vi "activateBtnIHM.vi"(8 "error in (no error)":errorcluster, 10 "State":T1(ring), 11 "References":T2) -> (0 "error out":errorcluster)   [LabVIEW 2023]
uses:
  referencesBtns.ctl
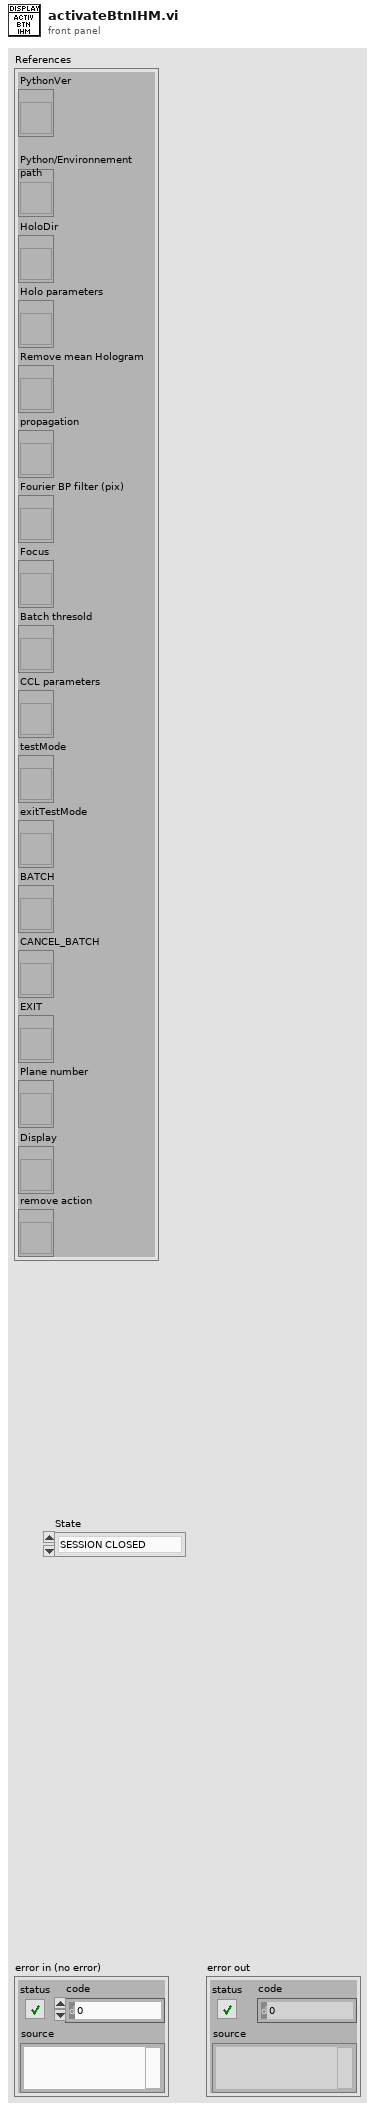
[diagram p1: front panel]
types:
  T1 = enum16{"SESSION CLOSED", "WAIT", "TEST WAIT", "TEST IN PROGESS", "BATCH IN PROGRESS"}
  T2 = typedef "referencesBtns.ctl" = cluster{"PythonVer":refnum<vi>, "Python/Environnement\npath":refnum<vi>, "HoloDir":refnum<vi>, "Holo parameters":refnum<vi>, "Remove mean Hologram":refnum<vi>, "propagation":refnum<vi>, "Fourier BP filter (pix)":refnum<vi>, "Focus":refnum<vi>, "Batch thresold ":refnum<vi>, "CCL parameters":refnum<vi>, "testMode":refnum<vi>, "exitTestMode":refnum<vi>, "BATCH":refnum<vi>, "CANCEL_BATCH":refnum<vi>, "EXIT":refnum<vi>, "Plane number":refnum<vi>, "Display":refnum<vi>, "remove action":refnum<vi>}
  T3 = enum16{"HOLOGRAM", "XY PLANE NUMBER....", "XY MAX PLANE", "XY SUM PLANE", "XZ MAX PLANE", "XZ SUM PLANE", "YZ MAX PLANE", "YZ SUM PLANE"}
  T4 = enum8{"Enabled", "Disabled", "Disabled and Grayed Out"}
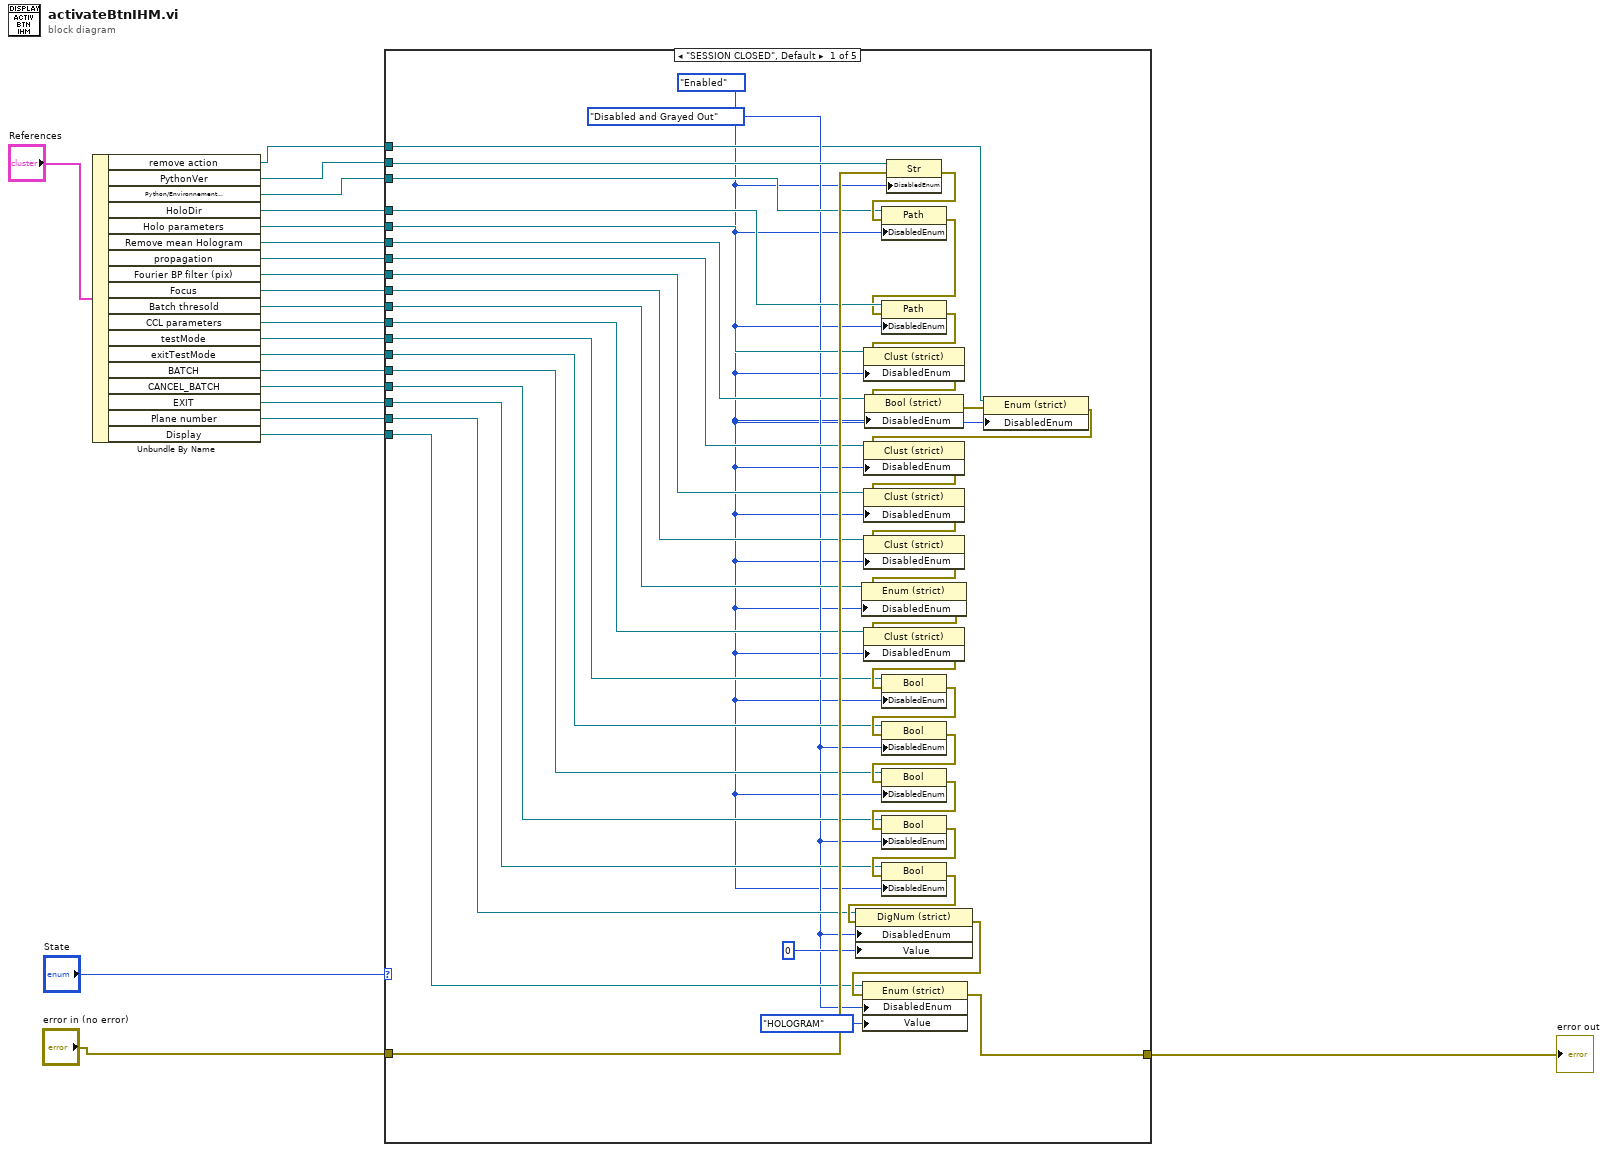
[diagram p0: block diagram]
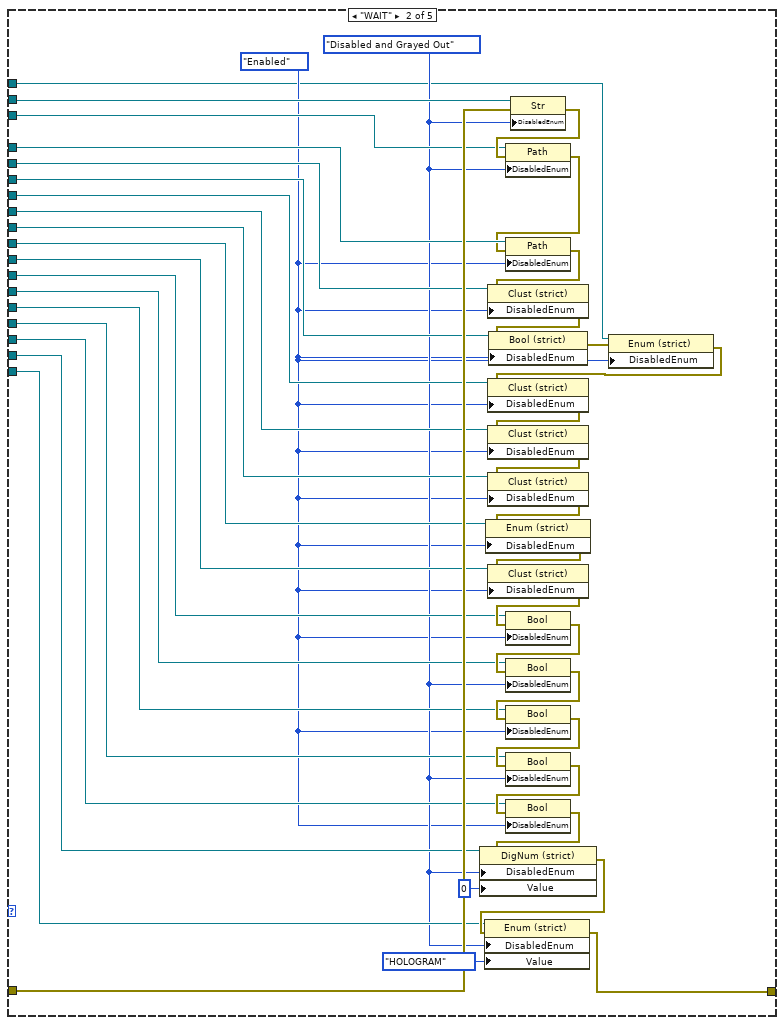
[diagram p2: hidden frame]
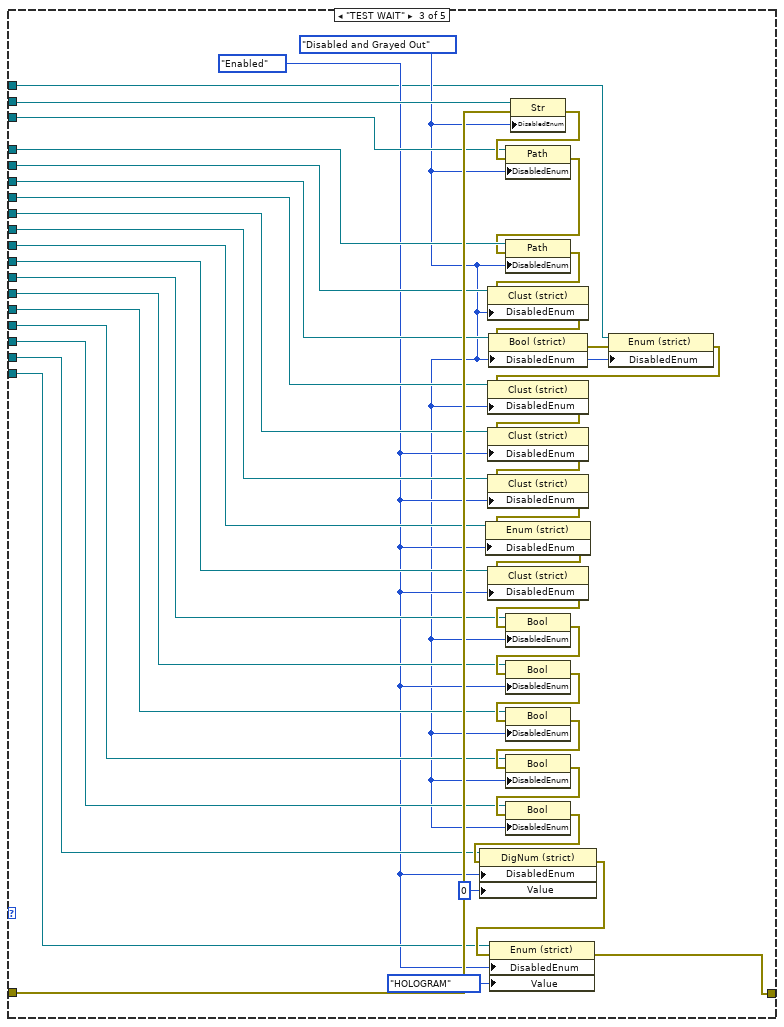
[diagram p3: hidden frame]
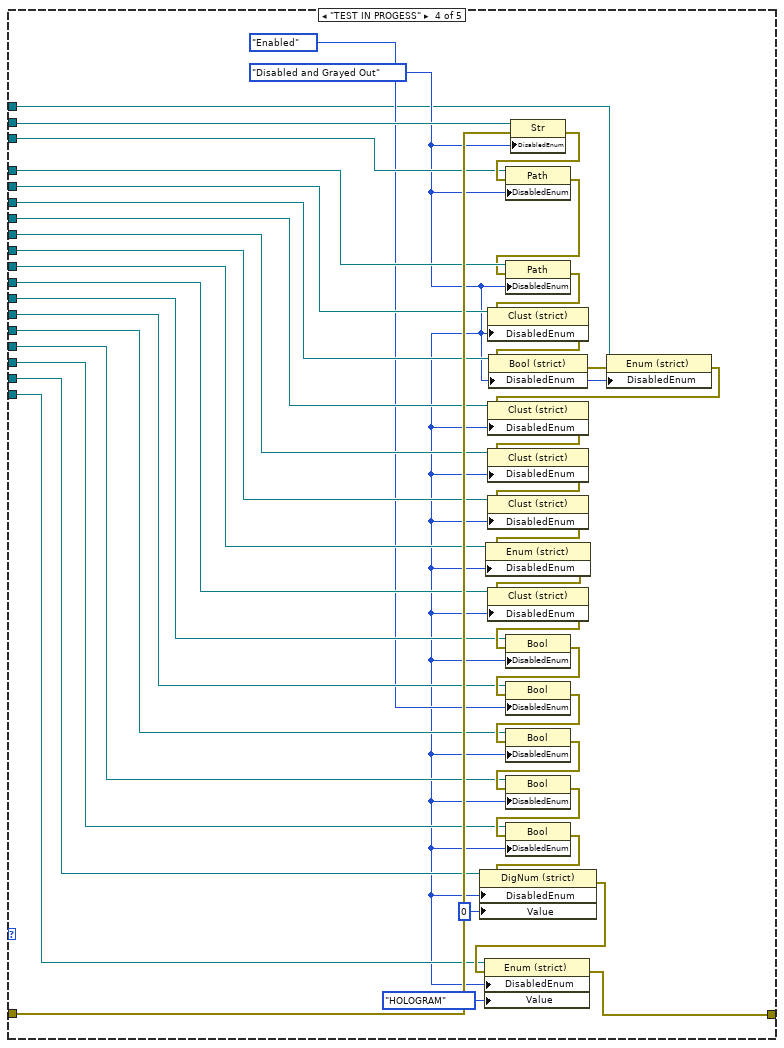
[diagram p4: hidden frame]
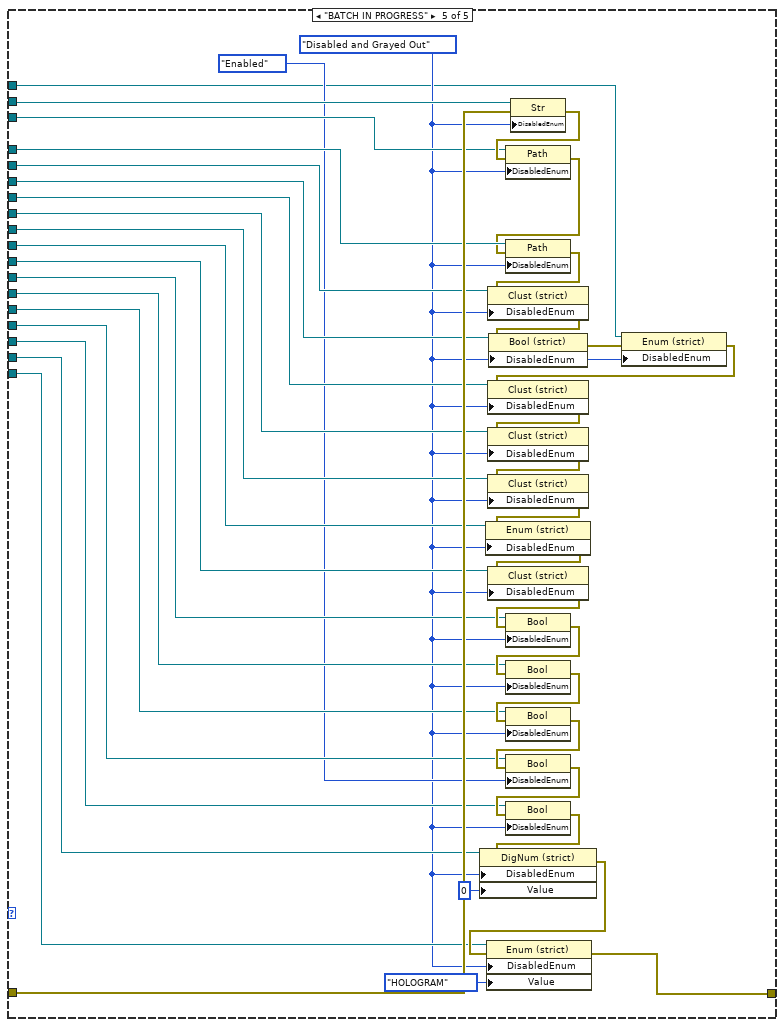
[diagram p5: hidden frame]
diagram:
  n1 = Unbundle By Name("References") -> ("remove action"=w1:refnum<vi>, "PythonVer"=w19:refnum<vi>, "Python/Environnement\npath"=w18:refnum<vi>, "HoloDir"=w17:refnum<vi>, "Holo parameters"=w16:refnum<vi>, "Remove mean Hologram"=w15:refnum<vi>, "propagation"=w14:refnum<vi>, "Fourier BP filter (pix)"=w13:refnum<vi>, "Focus"=w12:refnum<vi>, "Batch thresold"=w11:refnum<vi>, "CCL parameters"=w10:refnum<vi>, "testMode"=w9:refnum<vi>, "exitTestMode"=w8:refnum<vi>, "BATCH"=w7:refnum<vi>, "CANCEL_BATCH"=w6:refnum<vi>, "EXIT"=w5:refnum<vi>, "Plane number"=w4:refnum<vi>, "Display"=w2:refnum<vi>)
  n2 = case shown="\"SESSION CLOSED\", Default" "State" {
    tunnel: [w32 w73 w114 w154 w195] -> w21
    tunnel: "error in (no error)" -> [w62 w103 w144 w185 w226]
    tunnel: w19 -> [w63 w104 w145 w186 w227]
    tunnel: w18 -> [w48 w89 w130 w171 w212]
    tunnel: w17 -> [w47 w88 w129 w170 w211]
    tunnel: w16 -> [w46 w87 w128 w169 w210]
    tunnel: w15 -> [w45 w86 w127 w168 w209]
    tunnel: w14 -> [w44 w85 w126 w167 w208]
    tunnel: w13 -> [w43 w84 w125 w166 w207]
    tunnel: w12 -> [w42 w83 w124 w165 w206]
    tunnel: w11 -> [w41 w82 w123 w164 w205]
    tunnel: w10 -> [w40 w81 w122 w163 w204]
    tunnel: w9 -> [w39 w80 w121 w162 w203]
    tunnel: w8 -> [w38 w79 w120 w161 w202]
    tunnel: w7 -> [w37 w78 w119 w160 w201]
    tunnel: w6 -> [w36 w77 w118 w159 w200]
    tunnel: w5 -> [w35 w76 w117 w158 w199]
    tunnel: w4 -> [w34 w75 w116 w157 w198]
    tunnel: w2 -> [w31 w72 w113 w153 w194]
    tunnel: w1 -> [w24 w64 w105 w146 w188]
    frame "SESSION CLOSED", Default {
      w28 = T4."Disabled and Grayed Out" ("Disabled")
      w23 = T4."Enabled" ("Disabled")
      n3 = property class="Str"(reference=w63, error in=w62, "DisabledEnum"=w23) -> (error out=w61:errorcluster)  [unwired: 1 out]
      n4 = property class="Path"(reference=w48, error in=w61, "DisabledEnum"=w23) -> (error out=w27:errorcluster)  [unwired: 1 out]
      n5 = property class="Path"(reference=w47, error in=w27, "DisabledEnum"=w23) -> (error out=w60:errorcluster)  [unwired: 1 out]
      n6 = property class="Clust (strict)"(reference=w46, error in=w60, "DisabledEnum"=w23) -> (error out=w59:errorcluster)  [unwired: 1 out]
      n7 = property class="Bool (strict)"(reference=w45, error in=w59, "DisabledEnum"=w23) -> (error out=w26:errorcluster)  [unwired: 1 out]
      n8 = property class="Enum (strict)"(reference=w24, error in=w26, "DisabledEnum"=w23) -> (error out=w25:errorcluster)  [unwired: 1 out]
      n9 = property class="Clust (strict)"(reference=w44, error in=w25, "DisabledEnum"=w23) -> (error out=w58:errorcluster)  [unwired: 1 out]
      n10 = property class="Clust (strict)"(reference=w43, error in=w58, "DisabledEnum"=w23) -> (error out=w57:errorcluster)  [unwired: 1 out]
      n11 = property class="Clust (strict)"(reference=w42, error in=w57, "DisabledEnum"=w23) -> (error out=w56:errorcluster)  [unwired: 1 out]
      n12 = property class="Enum (strict)"(reference=w41, error in=w56, "DisabledEnum"=w23) -> (error out=w49:errorcluster)  [unwired: 1 out]
      n13 = property class="Clust (strict)"(reference=w40, error in=w49, "DisabledEnum"=w23) -> (error out=w50:errorcluster)  [unwired: 1 out]
      n14 = property class="Bool"(reference=w39, error in=w50, "DisabledEnum"=w23) -> (error out=w51:errorcluster)  [unwired: 1 out]
      n15 = property class="Bool"(reference=w38, error in=w51, "DisabledEnum"=w28) -> (error out=w53:errorcluster)  [unwired: 1 out]
      n16 = property class="Bool"(reference=w37, error in=w53, "DisabledEnum"=w23) -> (error out=w52:errorcluster)  [unwired: 1 out]
      n17 = property class="Bool"(reference=w36, error in=w52, "DisabledEnum"=w28) -> (error out=w54:errorcluster)  [unwired: 1 out]
      n18 = property class="Bool"(reference=w35, error in=w54, "DisabledEnum"=w23) -> (error out=w55:errorcluster)  [unwired: 1 out]
      n19 = property class="DigNum (strict)"(reference=w34, error in=w55, "DisabledEnum"=w28, "Value"=u16 0) -> (error out=w33:errorcluster)  [unwired: 1 out]
      n20 = property class="Enum (strict)"(reference=w31, error in=w33, "DisabledEnum"=w28, "Value"=T3."HOLOGRAM") -> (error out=w32:errorcluster)  [unwired: 1 out]
    }
    frame "WAIT" {
      w71 = T4."Disabled and Grayed Out" ("Disabled")
      w65 = T4."Enabled" ("Disabled")
      n21 = property class="Str"(reference=w104, error in=w103, "DisabledEnum"=w71) -> (error out=w102:errorcluster)  [unwired: 1 out]
      n22 = property class="Path"(reference=w89, error in=w102, "DisabledEnum"=w71) -> (error out=w68:errorcluster)  [unwired: 1 out]
      n23 = property class="Path"(reference=w88, error in=w68, "DisabledEnum"=w65) -> (error out=w101:errorcluster)  [unwired: 1 out]
      n24 = property class="Clust (strict)"(reference=w87, error in=w101, "DisabledEnum"=w65) -> (error out=w100:errorcluster)  [unwired: 1 out]
      n25 = property class="Bool (strict)"(reference=w86, error in=w100, "DisabledEnum"=w65) -> (error out=w67:errorcluster)  [unwired: 1 out]
      n26 = property class="Enum (strict)"(reference=w64, error in=w67, "DisabledEnum"=w65) -> (error out=w66:errorcluster)  [unwired: 1 out]
      n27 = property class="Clust (strict)"(reference=w85, error in=w66, "DisabledEnum"=w65) -> (error out=w99:errorcluster)  [unwired: 1 out]
      n28 = property class="Clust (strict)"(reference=w84, error in=w99, "DisabledEnum"=w65) -> (error out=w98:errorcluster)  [unwired: 1 out]
      n29 = property class="Clust (strict)"(reference=w83, error in=w98, "DisabledEnum"=w65) -> (error out=w97:errorcluster)  [unwired: 1 out]
      n30 = property class="Enum (strict)"(reference=w82, error in=w97, "DisabledEnum"=w65) -> (error out=w90:errorcluster)  [unwired: 1 out]
      n31 = property class="Clust (strict)"(reference=w81, error in=w90, "DisabledEnum"=w65) -> (error out=w91:errorcluster)  [unwired: 1 out]
      n32 = property class="Bool"(reference=w80, error in=w91, "DisabledEnum"=w65) -> (error out=w92:errorcluster)  [unwired: 1 out]
      n33 = property class="Bool"(reference=w79, error in=w92, "DisabledEnum"=w71) -> (error out=w94:errorcluster)  [unwired: 1 out]
      n34 = property class="Bool"(reference=w78, error in=w94, "DisabledEnum"=w65) -> (error out=w93:errorcluster)  [unwired: 1 out]
      n35 = property class="Bool"(reference=w77, error in=w93, "DisabledEnum"=w71) -> (error out=w95:errorcluster)  [unwired: 1 out]
      n36 = property class="Bool"(reference=w76, error in=w95, "DisabledEnum"=w65) -> (error out=w96:errorcluster)  [unwired: 1 out]
      n37 = property class="DigNum (strict)"(reference=w75, error in=w96, "DisabledEnum"=w71, "Value"=u16 0) -> (error out=w74:errorcluster)  [unwired: 1 out]
      n38 = property class="Enum (strict)"(reference=w72, error in=w74, "DisabledEnum"=w71, "Value"=T3."HOLOGRAM") -> (error out=w73:errorcluster)  [unwired: 1 out]
    }
    frame "TEST WAIT" {
      w108 = T4."Disabled and Grayed Out" ("Disabled")
      w112 = T4."Enabled" ("Disabled")
      n39 = property class="Str"(reference=w145, error in=w144, "DisabledEnum"=w108) -> (error out=w143:errorcluster)  [unwired: 1 out]
      n40 = property class="Path"(reference=w130, error in=w143, "DisabledEnum"=w108) -> (error out=w109:errorcluster)  [unwired: 1 out]
      n41 = property class="Path"(reference=w129, error in=w109, "DisabledEnum"=w108) -> (error out=w142:errorcluster)  [unwired: 1 out]
      n42 = property class="Clust (strict)"(reference=w128, error in=w142, "DisabledEnum"=w108) -> (error out=w141:errorcluster)  [unwired: 1 out]
      n43 = property class="Bool (strict)"(reference=w127, error in=w141, "DisabledEnum"=w108) -> (error out=w107:errorcluster)  [unwired: 1 out]
      n44 = property class="Enum (strict)"(reference=w105, error in=w107, "DisabledEnum"=w108) -> (error out=w106:errorcluster)  [unwired: 1 out]
      n45 = property class="Clust (strict)"(reference=w126, error in=w106, "DisabledEnum"=w108) -> (error out=w140:errorcluster)  [unwired: 1 out]
      n46 = property class="Clust (strict)"(reference=w125, error in=w140, "DisabledEnum"=w112) -> (error out=w139:errorcluster)  [unwired: 1 out]
      n47 = property class="Clust (strict)"(reference=w124, error in=w139, "DisabledEnum"=w112) -> (error out=w138:errorcluster)  [unwired: 1 out]
      n48 = property class="Enum (strict)"(reference=w123, error in=w138, "DisabledEnum"=w112) -> (error out=w131:errorcluster)  [unwired: 1 out]
      n49 = property class="Clust (strict)"(reference=w122, error in=w131, "DisabledEnum"=w112) -> (error out=w132:errorcluster)  [unwired: 1 out]
      n50 = property class="Bool"(reference=w121, error in=w132, "DisabledEnum"=w108) -> (error out=w133:errorcluster)  [unwired: 1 out]
      n51 = property class="Bool"(reference=w120, error in=w133, "DisabledEnum"=w112) -> (error out=w135:errorcluster)  [unwired: 1 out]
      n52 = property class="Bool"(reference=w119, error in=w135, "DisabledEnum"=w108) -> (error out=w134:errorcluster)  [unwired: 1 out]
      n53 = property class="Bool"(reference=w118, error in=w134, "DisabledEnum"=w108) -> (error out=w136:errorcluster)  [unwired: 1 out]
      n54 = property class="Bool"(reference=w117, error in=w136, "DisabledEnum"=w108) -> (error out=w137:errorcluster)  [unwired: 1 out]
      n55 = property class="DigNum (strict)"(reference=w116, error in=w137, "DisabledEnum"=w112, "Value"=u16 0) -> (error out=w115:errorcluster)  [unwired: 1 out]
      n56 = property class="Enum (strict)"(reference=w113, error in=w115, "DisabledEnum"=w112, "Value"=T3."HOLOGRAM") -> (error out=w114:errorcluster)  [unwired: 1 out]
    }
    frame "TEST IN PROGESS" {
      w148 = T4."Disabled and Grayed Out" ("Disabled")
      n57 = property class="Str"(reference=w186, error in=w185, "DisabledEnum"=w148) -> (error out=w184:errorcluster)  [unwired: 1 out]
      n58 = property class="Path"(reference=w171, error in=w184, "DisabledEnum"=w148) -> (error out=w150:errorcluster)  [unwired: 1 out]
      n59 = property class="Path"(reference=w170, error in=w150, "DisabledEnum"=w148) -> (error out=w183:errorcluster)  [unwired: 1 out]
      n60 = property class="Clust (strict)"(reference=w169, error in=w183, "DisabledEnum"=w148) -> (error out=w182:errorcluster)  [unwired: 1 out]
      n61 = property class="Bool (strict)"(reference=w168, error in=w182, "DisabledEnum"=w148) -> (error out=w149:errorcluster)  [unwired: 1 out]
      n62 = property class="Enum (strict)"(reference=w146, error in=w149, "DisabledEnum"=w148) -> (error out=w147:errorcluster)  [unwired: 1 out]
      n63 = property class="Clust (strict)"(reference=w167, error in=w147, "DisabledEnum"=w148) -> (error out=w181:errorcluster)  [unwired: 1 out]
      n64 = property class="Clust (strict)"(reference=w166, error in=w181, "DisabledEnum"=w148) -> (error out=w180:errorcluster)  [unwired: 1 out]
      n65 = property class="Clust (strict)"(reference=w165, error in=w180, "DisabledEnum"=w148) -> (error out=w179:errorcluster)  [unwired: 1 out]
      n66 = property class="Enum (strict)"(reference=w164, error in=w179, "DisabledEnum"=w148) -> (error out=w172:errorcluster)  [unwired: 1 out]
      n67 = property class="Clust (strict)"(reference=w163, error in=w172, "DisabledEnum"=w148) -> (error out=w173:errorcluster)  [unwired: 1 out]
      n68 = property class="Bool"(reference=w162, error in=w173, "DisabledEnum"=w148) -> (error out=w174:errorcluster)  [unwired: 1 out]
      n69 = property class="Bool"(reference=w161, error in=w174, "DisabledEnum"=T4."Enabled" ("Disabled")) -> (error out=w176:errorcluster)  [unwired: 1 out]
      n70 = property class="Bool"(reference=w160, error in=w176, "DisabledEnum"=w148) -> (error out=w175:errorcluster)  [unwired: 1 out]
      n71 = property class="Bool"(reference=w159, error in=w175, "DisabledEnum"=w148) -> (error out=w177:errorcluster)  [unwired: 1 out]
      n72 = property class="Bool"(reference=w158, error in=w177, "DisabledEnum"=w148) -> (error out=w178:errorcluster)  [unwired: 1 out]
      n73 = property class="DigNum (strict)"(reference=w157, error in=w178, "DisabledEnum"=w148, "Value"=u16 0) -> (error out=w155:errorcluster)  [unwired: 1 out]
      n74 = property class="Enum (strict)"(reference=w153, error in=w155, "DisabledEnum"=w148, "Value"=T3."HOLOGRAM") -> (error out=w154:errorcluster)  [unwired: 1 out]
    }
    frame "BATCH IN PROGRESS" {
      w189 = T4."Disabled and Grayed Out" ("Disabled")
      n75 = property class="Str"(reference=w227, error in=w226, "DisabledEnum"=w189) -> (error out=w225:errorcluster)  [unwired: 1 out]
      n76 = property class="Path"(reference=w212, error in=w225, "DisabledEnum"=w189) -> (error out=w191:errorcluster)  [unwired: 1 out]
      n77 = property class="Path"(reference=w211, error in=w191, "DisabledEnum"=w189) -> (error out=w224:errorcluster)  [unwired: 1 out]
      n78 = property class="Clust (strict)"(reference=w210, error in=w224, "DisabledEnum"=w189) -> (error out=w223:errorcluster)  [unwired: 1 out]
      n79 = property class="Bool (strict)"(reference=w209, error in=w223, "DisabledEnum"=w189) -> (error out=w190:errorcluster)  [unwired: 1 out]
      n80 = property class="Enum (strict)"(reference=w188, error in=w190, "DisabledEnum"=w189) -> (error out=w187:errorcluster)  [unwired: 1 out]
      n81 = property class="Clust (strict)"(reference=w208, error in=w187, "DisabledEnum"=w189) -> (error out=w222:errorcluster)  [unwired: 1 out]
      n82 = property class="Clust (strict)"(reference=w207, error in=w222, "DisabledEnum"=w189) -> (error out=w221:errorcluster)  [unwired: 1 out]
      n83 = property class="Clust (strict)"(reference=w206, error in=w221, "DisabledEnum"=w189) -> (error out=w220:errorcluster)  [unwired: 1 out]
      n84 = property class="Enum (strict)"(reference=w205, error in=w220, "DisabledEnum"=w189) -> (error out=w213:errorcluster)  [unwired: 1 out]
      n85 = property class="Clust (strict)"(reference=w204, error in=w213, "DisabledEnum"=w189) -> (error out=w214:errorcluster)  [unwired: 1 out]
      n86 = property class="Bool"(reference=w203, error in=w214, "DisabledEnum"=w189) -> (error out=w215:errorcluster)  [unwired: 1 out]
      n87 = property class="Bool"(reference=w202, error in=w215, "DisabledEnum"=w189) -> (error out=w217:errorcluster)  [unwired: 1 out]
      n88 = property class="Bool"(reference=w201, error in=w217, "DisabledEnum"=w189) -> (error out=w216:errorcluster)  [unwired: 1 out]
      n89 = property class="Bool"(reference=w200, error in=w216, "DisabledEnum"=T4."Enabled" ("Disabled")) -> (error out=w218:errorcluster)  [unwired: 1 out]
      n90 = property class="Bool"(reference=w199, error in=w218, "DisabledEnum"=w189) -> (error out=w219:errorcluster)  [unwired: 1 out]
      n91 = property class="DigNum (strict)"(reference=w198, error in=w219, "DisabledEnum"=w189, "Value"=u16 0) -> (error out=w196:errorcluster)  [unwired: 1 out]
      n92 = property class="Enum (strict)"(reference=w194, error in=w196, "DisabledEnum"=w189, "Value"=T3."HOLOGRAM") -> (error out=w195:errorcluster)  [unwired: 1 out]
    }
  }
  "error out" <- w21
